vi "insert_double.vi"(6 "Time Stamp":timestamp, 8 "error in (no error)":errorcluster, 9 "Value":dbl, 10 "path table:column":string, 11 "Data.PG in":refnum<class "Data.PG.lvclass">=refnum) -> (0 "error out":errorcluster, 3 "Data.PG out":refnum<class "Data.PG.lvclass">)   [LabVIEW 2020, in "Data.PG.lvclass"]
uses:
  Data.PG.lvclass
  <vilib>/JDP Science/PostgreSQL Library/Connection/PQ Connection.lvclass
  Data/Typedefs/Operation--enum.ctl
  Data.PG.lvclass/Data.PG.ctl
  <vilib>/JDP Science/PostgreSQL Library/Result/PQ Result.lvclass/PQ Result.ctl
  <vilib>/JDP Science/PostgreSQL Library/Connection/Execute Command (2D string results).vi
  <vilib>/JDP Science/PostgreSQL Library/Result/Clear.vi
  <vilib>/JDP Science/PostgreSQL Library/Connection/Execute Command (Result).vi
  <vilib>/JDP Science/PostgreSQL Library/Connection/Execute (Return first result with rows).vi
  <vilib>/JDP Science/PostgreSQL Library/Connection/Single Command with parameters.vi
  <vilib>/JDP Science/PostgreSQL Library/Result/Get all results as 2D strings array.vi
  Data/Data.lvclass
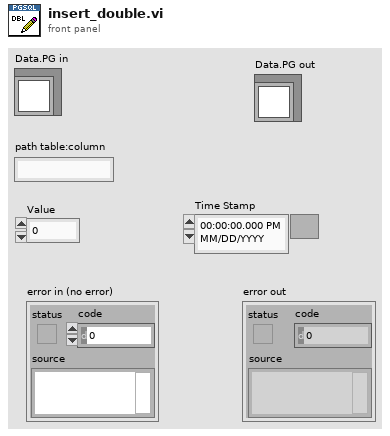
[diagram p1: front panel]
types:
  T1 = typedef "Data.lvclass/Operation--enum.ctl" = enum16{"Read", "Write", "Write + Append"}
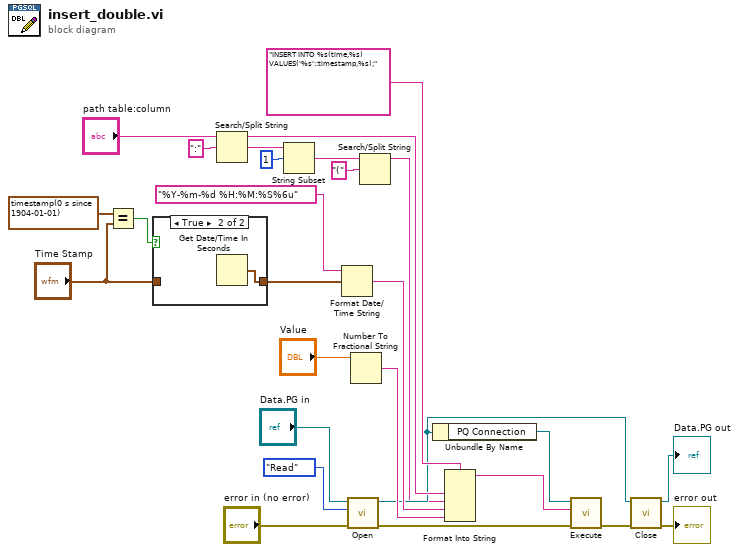
[diagram p0: block diagram]
diagram:
  n1 = Equal?(x=timestamp(0 s since 1904-01-01), y="Time Stamp") -> (x = y?=w4:bool)
  n2 = case shown="True" w4 {
    tunnel: [w28 w29] -> w1
    tunnel: "Time Stamp" -> [w28 _]
    frame False {
    }
    frame True {
      n3 = Get Date/Time In Seconds() -> (seconds since 1Jan1904=w29:timestamp)
    }
  }
  n4 = Search/Split String(string="path table:column", search string/char (-)=":") -> (substring before match=w24:string, match + rest of string=w23:string)  [unwired: 1 in, 1 out]
  n5 = String Subset(string=w23, offset (0)=1) -> (substring=w7:string)  [unwired: 1 in]
  n6 = Format Date/Time String(time format string (%c)="%Y-%m-%d %H:%M:%S%6u", seconds (now)=w1) -> (date/time string=w20:string)  [unwired: 1 in]
  n7 = call-dynamic "Open.vi"("error in (no error)"="error in (no error)", "Operation"=Operation--enum."Read", "Data.PG in"="Data.PG in") -> ("error out"=w14:errorcluster, "Data.PG out"=w9:refnum<class "Data.PG.lvclass">)  [unwired: 7 in]
  n8 = Number To Fractional String(number="Value") -> (F-format string=w18:string)  [unwired: 3 in]
  n9 = Search/Split String(string=w7, search string/char (-)="(") -> (substring before match=w6:string)  [unwired: 1 in, 2 out]
  n10 = Unbundle By Name(w9) -> ("PQ Connection"=w8:refnum<class "PQ Connection.lvclass">)
  n11 = Format Into String(format string="INSERT INTO %s(time,%s) VALUES('%s'::timestamp,%s);", w24, w6, w20, w18) -> (resulting string=w10:string)  [unwired: 2 in, 1 out]
  n12 = call-poly <vilib>:"Execute.vi"("error in (no error)"=w14, "SQL"=w10, "PQ Connection in"=w8) -> ("error out"=w13:errorcluster)  [unwired: 5 in, 3 out]
  n13 = call-dynamic "Close.vi"("error in (no error)"=w13, "Data.PG in"=w9) -> ("error out"=→"error out":errorcluster, "Data.PG out"=→"Data.PG out":refnum<class "Data.PG.lvclass">)  [unwired: 8 in]
